vi "Msg.vi"(7 "jettl in":refnum<class "jettl.lvclass">, 11 "Pop Up Msg Strategy in":refnum<class "Pop Up Msg Strategy.lvclass">) -> (5 "jettl out":refnum<class "jettl.lvclass">)   [LabVIEW 2021, in "Pop Up.lvlib" / "Pop Up Msg Strategy.lvclass"]
uses:
  Pop Up Msg Strategy.lvclass
  Pop Up Msg Strategy.lvclass/Pop Up Msg Strategy.ctl
  Pop Up/Pop Up.lvclass
  jettl/jettl/jettl/jettl.lvclass
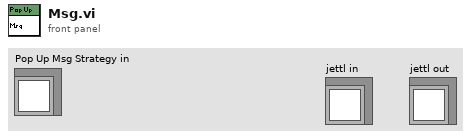
[diagram p1: front panel]
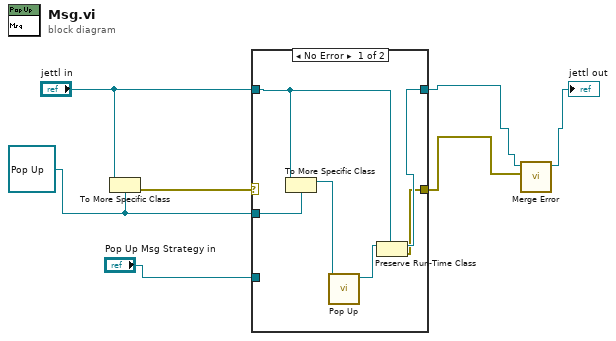
[diagram p0: block diagram]
diagram:
  w5 = refnum<class "Pop Up.lvclass"> refnum ("Pop Up.lvlib:Pop Up.lvclass")
  n1 = To More Specific Class(target class=w5, reference="jettl in") -> (error out=w7:errorcluster)  [unwired: 1 in, 1 out]
  n2 = case shown="No Error" w7 {
    selector: w7 -> [_ w14]
    tunnel: [w9 w15] -> w4
    tunnel: "jettl in" -> [w11 w15]
    tunnel: w5 -> [w13 _]
    tunnel: "Pop Up Msg Strategy in" -> [_ _]
    tunnel: [w8 w14] -> w3
    frame No Error {
      n3 = To More Specific Class(target class=w13, reference=w11) -> (specific class reference=w12:refnum<class "Pop Up.lvclass">)  [unwired: 1 in, 1 out]
      n4 = call-dynamic "Pop Up.vi"("Pop Up in"=w12) -> ("Pop Up out"=w10:refnum<class "Pop Up.lvclass">)  [unwired: 10 in]
      n5 = Preserve Run-Time Class(object in=w10, 2:w11) -> (object out=w9:refnum<class "jettl.lvclass">, error out=w8:errorcluster)  [unwired: 1 in]
    }
    frame Error {
    }
  }
  n6 = call-dynamic "Merge Error.vi"("Error"=w3, "Merge Error in"=w4) -> ("Merge Error out"=→"jettl out":refnum<class "jettl.lvclass">)  [unwired: 9 in]
